vi "WSVCAP SHL Host TL I2C Write - Multiple Device - Common Data.vi"(0 "Sub Address":u8=20 format="%.0x", 3 "FPGA":T1, 5 "Data Out [U8]":u8=20 format="%.0x", 11 "error in":errorcluster, 12 "Log (T)":bool=TRUE, 13 "DUT Mask Array (All)":bool[](array[boolean])=[TRUE, TRUE, TRUE, TRUE, TRUE, TRUE, TRUE, TRUE, TRUE, TRUE, TRUE, TRUE, TRUE, TRUE, TRUE, TRUE, TRUE, TRUE, TRUE, TRUE, TRUE, TRUE, TRUE, TRUE, TRUE, TRUE, TRUE, TRUE, TRUE, TRUE, TRUE, TRUE, TRUE, TRUE, TRUE, TRUE, TRUE, TRUE, TRUE, TRUE, TRUE, TRUE, TRUE, TRUE, TRUE, TRUE, TRUE, TRUE, TRUE, TRUE, TRUE, TRUE, TRUE, TRUE, TRUE, TRUE, TRUE, TRUE, TRUE, TRUE, TRUE, TRUE, TRUE, TRUE], 14 "DUT Mask Mode (All)":T2=enum."All") -> (15 "error out":errorcluster)   [LabVIEW 2017]
uses:
  Type Defs/WSVCAP SHL I2C DUT Mask Mode Enum.ctl
  Type Defs/WSVCAP SHL FPGA Enum.ctl
panel:
  out "Socket Mask [U64]":u64 format="%06x"
  out "C1 Data Out":u8[](array[numeric]) format="%.0x"
  # "DUT 01"
  # "DUT 02"
  # "DUT 03"
  # "DUT 04"
  # "DUT 05"
  # "DUT 06"
  # "DUT 07"
  # "DUT 08"
  # "DUT 09"
  # "DUT 10"
  # "DUT 11"
  # "DUT 12"
  # "DUT 13"
  # "DUT 14"
  # "DUT 15"
  # "DUT 16"
  # "DUT 17"
  # "DUT 18"
  # "DUT 19"
  # "DUT 20"
  # "DUT 21"
  # "DUT 22"
  # "DUT 23"
  # "DUT 24"
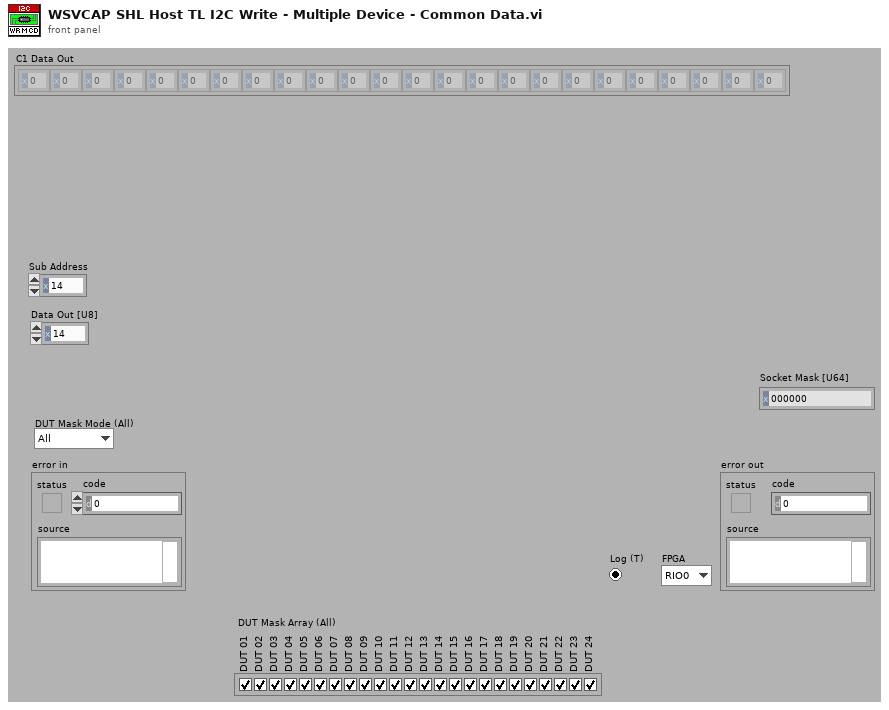
[diagram p1: front panel]
types:
  T1 = typedef "WSVCAP SHL FPGA Enum.ctl" = enum16{"RIO0", "RIO1"}
  T2 = typedef "WSVCAP SHL I2C DUT Mask Mode Enum.ctl" = enum16{"Custom", "All"}
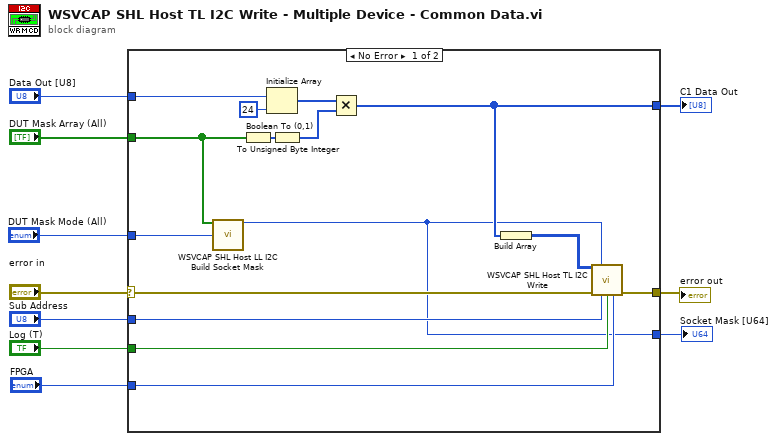
[diagram p0: block diagram]
diagram:
  n1 = case shown="No Error" "error in" {
    selector: "error in" -> [w20 w26]
    tunnel: [w25 w26] -> w10
    tunnel: "Sub Address" -> [w18 _]
    tunnel: "Data Out [U8]" -> [w22 _]
    tunnel: [w21 _] -> w6
    tunnel: [w14 _] -> w5
    tunnel: "DUT Mask Array (All)" -> [w12 _]
    tunnel: "Log (T)" -> [w19 _]
    tunnel: "DUT Mask Mode (All)" -> [w17 _]
    tunnel: "FPGA" -> [w16 _]
    frame No Error {
      n2 = call "WSVCAP SHL Host LL I2C Build Socket Mask.vi"("DUT Mask Array (All)"=w12, "DUT Mask Mode (Custom)"=w17) -> ("Socket Mask Set [U64]"=w14:u64)  [unwired: 13 in]
      n3 = Boolean To (0,1)(Boolean=w12) -> (0, 1=w23:i16[])
      n4 = Initialize Array(w22, 24 ("dimension size")) -> (w15:u8[])
      n5 = To Unsigned Byte Integer(number=w23) -> (unsigned 8bit integer=w13:u8[])
      n6 = Multiply(x=w15, y=w13) -> (x*y=w21:u8[])
      n7 = Build Array(w21) -> (w24:u8[][])
      n8 = call "WSVCAP SHL Host TL I2C Write.vi"("C Data Out"=w24, "Socket Mask [U64]"=w14, "error in"=w20, "Sub Address"=w18, "Log (T)"=w19, "FPGA"=w16) -> ("error out"=w25:errorcluster)  [unwired: 9 in]
    }
    frame Error {
    }
  }
  "error out" <- w10
  "C1 Data Out" <- w6
  "Socket Mask [U64]" <- w5
